vi "BluetoothHandler.vi"(11 "Queue":refnum<queue>) -> ()   [LabVIEW 2013, in "main.lvlib"]
uses:
  main.lvlib
  Controls/Enum Save Action Events.ctl
  C:/Users/Simon/SkyDrive/LabView/2013/DM2020/bin/medimatic_bt_receiver.dll
  bin/medimatic_bt_receiver.dll
panel:
  out "Present (s)":dbl
  out "Elapsed Time (s)":dbl
  out "Msg":string
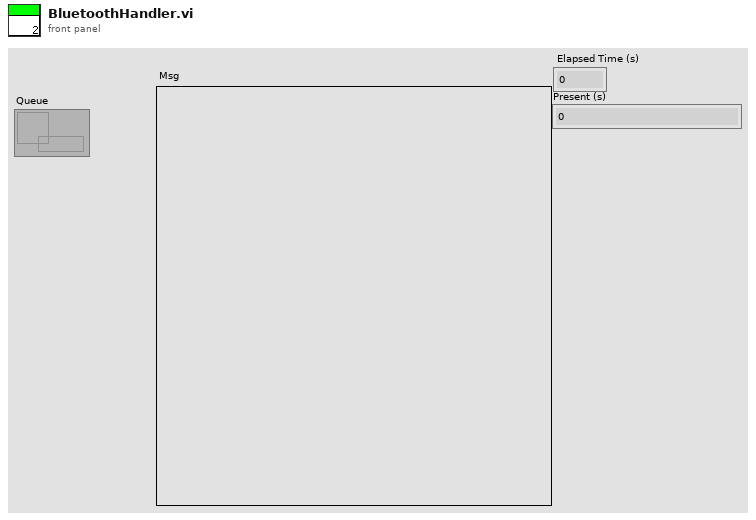
[diagram p1: front panel]
types:
  T1 = typedef "main.lvlib/Enum Save Action Events.ctl" = enum16{"LoadReportPath", "SaveReportPath", "Load Graph Path", "Save Graph Path", "LoadDataPath", "SaveDataPath", "Load Template Path", "Save Template Path", "Load PressureFactor", "Save PressureFactor", "Init", "Load Listbox", "Save Listbox", "LoadHospInfo", "SaveHospInfo", "Load DICOM Activation", "Save DICOM Activation", "LoadDICOMInfoWL", "SaveDICOMInfoWL", "LoadDICOMInfoPACS", "SaveDICOMInfoPACS", "Load ArmCalcMethod", "Save ArmCalcMethod", "LoadItemTags", "SaveItemTags", "LoadDICOMEncoding", "SaveDICOMEncoding", "LoadJournalType", "SaveJournalType", "LoadAcqFilterType", "SaveAcqFilterType", "Load Sequence", "Save Sequence", "Load Acquisition Mode", "Save Acquisition Mode", "Load General Settings", "Save General Settings", "Load Language", "Save Language", "Load Dicom Tags", "Save Dicom Tags", "Load BT Serial", "Save BT Serial", "Load BT License", "Save BT License"}
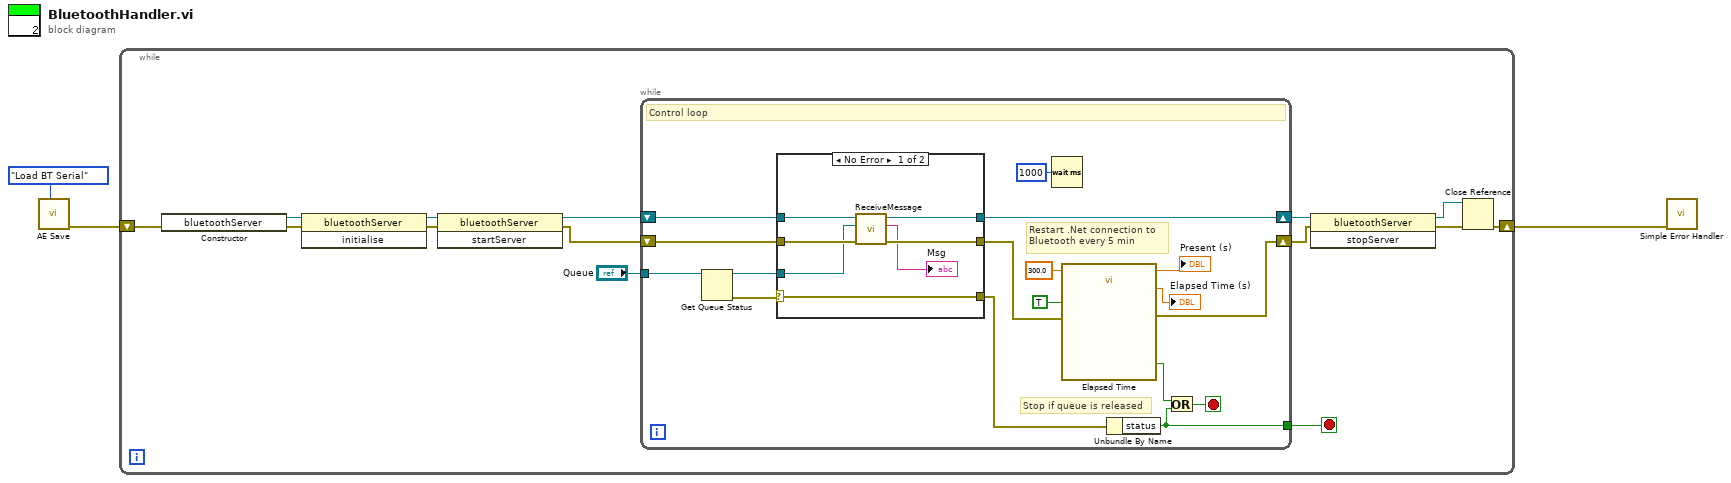
[diagram p0: block diagram]
diagram:
  n1 = call "AE Save.vi"("Action"=Enum_Save_Action_Events."Load BT Serial") -> ("error out"=w2:errorcluster)  [unwired: 8 in, 1 out]
  n2 = while {
    shift-right: [w6] -> w1
    shift-left: w2 -> [w7]
    stop <- w5 stop-if-true
    n3 = constructor class="bluetoothServer"(error in=w7) -> (reference out=w17:refnum<k24>, error out=w15:errorcluster)  [unwired: 2 in, 1 out]
    n4 = invoke class="bluetoothServer" method="initialise"(reference=w17, error in=w15) -> (reference out=w16:refnum<k24>, error out=w14:errorcluster)  [unwired: 1 in, 1 out]
    n5 = invoke class="bluetoothServer" method="startServer"(reference=w16, error in=w14) -> (reference out=w11:refnum<k24>, error out=w9:errorcluster)  [unwired: 1 in, 1 out]
    n6 = while {
      tunnel: "Queue" -> [w30]
      shift-right: [w33] -> w10
      shift-left: w11 -> [w34]
      shift-right: [w26] -> w4
      shift-left: w9 -> [w32]
      tunnel: [w20] -> w5
      stop <- w23 stop-if-true
      # "Restart .Net connection to\nBluetooth every 5 min"
      # "Stop if queue is released"
      # "Control loop"
      n7 = Get Queue Status(queue=w30) -> (queue out=w29:refnum<queue>, error out=w28:errorcluster)  [unwired: 2 in, 6 out]
      n8 = case shown="No Error" w28 {
        selector: w28 -> [w36 w44]
        tunnel: w34 -> [w41 w43]
        tunnel: [w40 w43] -> w33
        tunnel: w32 -> [w39 w42]
        tunnel: [w38 w42] -> w27
        tunnel: w29 -> [w37 _]
        tunnel: [w36 w44] -> w21
        frame No Error {
          n9 = call "ReceiveMessage.vi"("error in (no error)"=w39, "BT Queue"=w37, ".NET Refnum in"=w41) -> ("error out"=w38:errorcluster, "String"=→"Msg":string, ".NET Refnum out"=w40:refnum<k24>)  [unwired: 6 in]
        }
        frame Error {
        }
      }
      n10 = Wait (ms)(milliseconds to wait=1000) -> ()  [unwired: 1 out]
      n11 = call "Elapsed Time"("Time Target (s)"=300.0, "Auto Reset"=TRUE, "error in (no error)"=w27) -> ("Present (s)"=→"Present (s)":dbl, "Elapsed Time (s)"=→"Elapsed Time (s)":dbl, "Time has Elapsed"=w22:bool, "error out"=w26:errorcluster)  [unwired: 9 in, 4 out]
      n12 = Unbundle By Name(w21) -> ("status"=w20:bool)
      n13 = Or(x=w22, y=w20) -> (x .or. y?=w23:bool)
    }
    n14 = invoke class="bluetoothServer" method="stopServer"(reference=w10, error in=w4) -> (reference out=w12:refnum<k24>, error out=w13:errorcluster)  [unwired: 1 in, 1 out]
    n15 = Close Reference(reference=w12, error in (no error)=w13) -> (error out=w6:errorcluster)
  }
  n16 = call <vilib>:"Simple Error Handler.vi"("error in (no error)"=w1) -> ()  [unwired: 4 in, 5 out]
